vi "K-means Clustering.vi"() -> ()   [LabVIEW 2020]
doc: "The plots display firstly what a K-means algorithm would yield using three clusters. It is then shown what the effect of a bad initialization is on the classification process: By setting n_init to only 1 (default is 10), the amount of times that the algorithm will be run with different centroid seeds is reduced. The next plot displays what using eight clusters would deliver and finally the ground truth."
uses:
  <vilib>/Math Plots/3D Math Plots/3D Scatter/3D Scatter XCtrl/3D Scatter.xctl
  Model/Unsupervised/Cluster/KMeans/KMeans.lvclass
  C:/Users/cipop/TDF Dropbox/2_Technologies de France/1 - Services et Etudes/PLAIY/2 - DEV/PLAIYLAB/code/Model/Model.lvclass
  Model/Unsupervised/Cluster/KMeans/Controls/kmeans_params.ctl
  <vilib>/Math Plots/3D Math Plots/3D Plot/3D Plot Datatype/3D Plot Datatype.lvclass
  PLAIYDISPLAY/Display/_Controls/Style.ctl
  Model/Unsupervised/Cluster/KMeans/KMeans.vi
panel:
  in  "Local":T1
  out "3D Scatter":refnum<class "3D Plot Datatype.lvclass">[](xcontrol)
  out "error out":errorcluster
  in  "error in":errorcluster
  out "3D Scatter 4":refnum<class "3D Plot Datatype.lvclass">[](xcontrol)
  out "3D Scatter 3":refnum<class "3D Plot Datatype.lvclass">[](xcontrol)
  out "3D Scatter 2":refnum<class "3D Plot Datatype.lvclass">[](xcontrol)
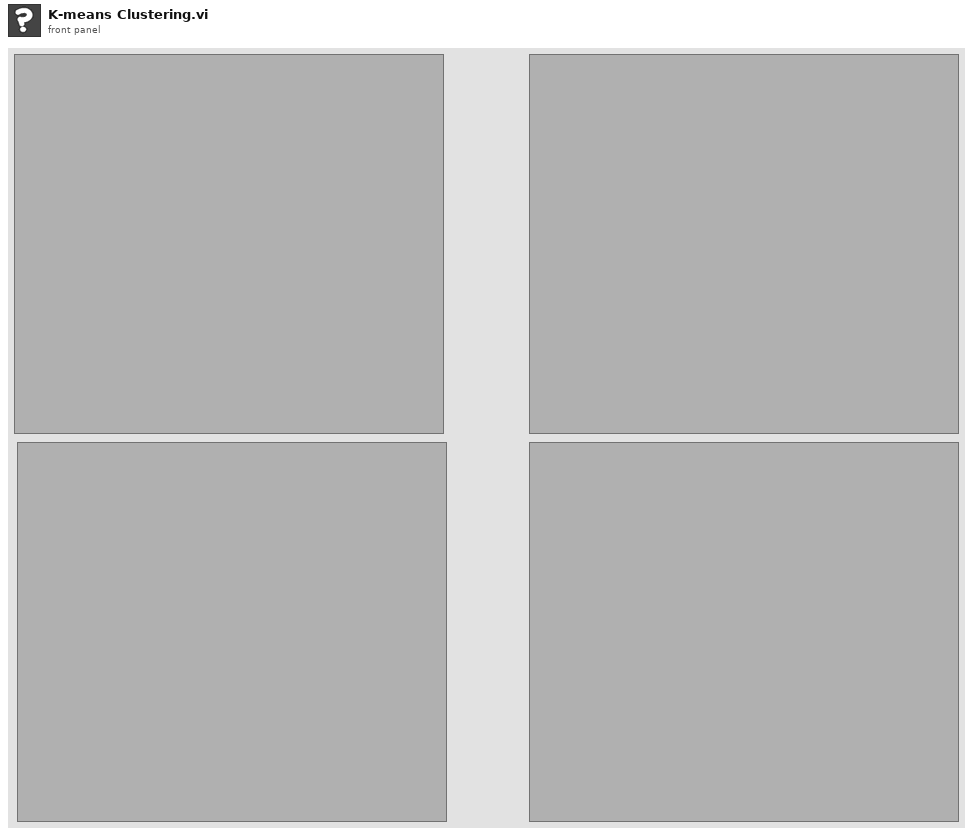
[diagram p1: front panel]
types:
  T1 = cluster{"X":dbl[][], "Y":dbl[], "KMeans":refnum<class "KMeans.lvclass">}
  T2 = typedef "Style.ctl" = enum16{"Empty circle", "Full circle", "Empty square", "Full square", "Cross"}
  T3 = cluster{"Parameter":cluster{"3D Plot":refnum<class "3D Plot Datatype.lvclass">[], "3D Scatter":refnum<vi>, "Data":cluster{"X":dbl[][], "Predict":dbl[][]}, "Display":cluster{"Choice":enum16{"All", "Train", "Test"}, "Indexe":cluster{"X":i32, "Y":i32, "Z":i32}}, "Point Property":cluster{"Style":T2, "Label Color":u32[]}}}
  T4 = typedef "kmeans_params.ctl" = cluster{"n_clusters":dbl, "init":cluster{"init_type":string, "init_list":dbl[][]}, "n_init":dbl, "max_iter":dbl, "tol":dbl, "verbose":dbl, "random_state":dbl, "copy_x":bool, "algorithm":string}
  T5 = typedef "kmeans_attributes.ctl" = cluster{"cluster_centers_":dbl[][], "labels_":dbl[], "inertia_":dbl, "n_iter_":dbl}
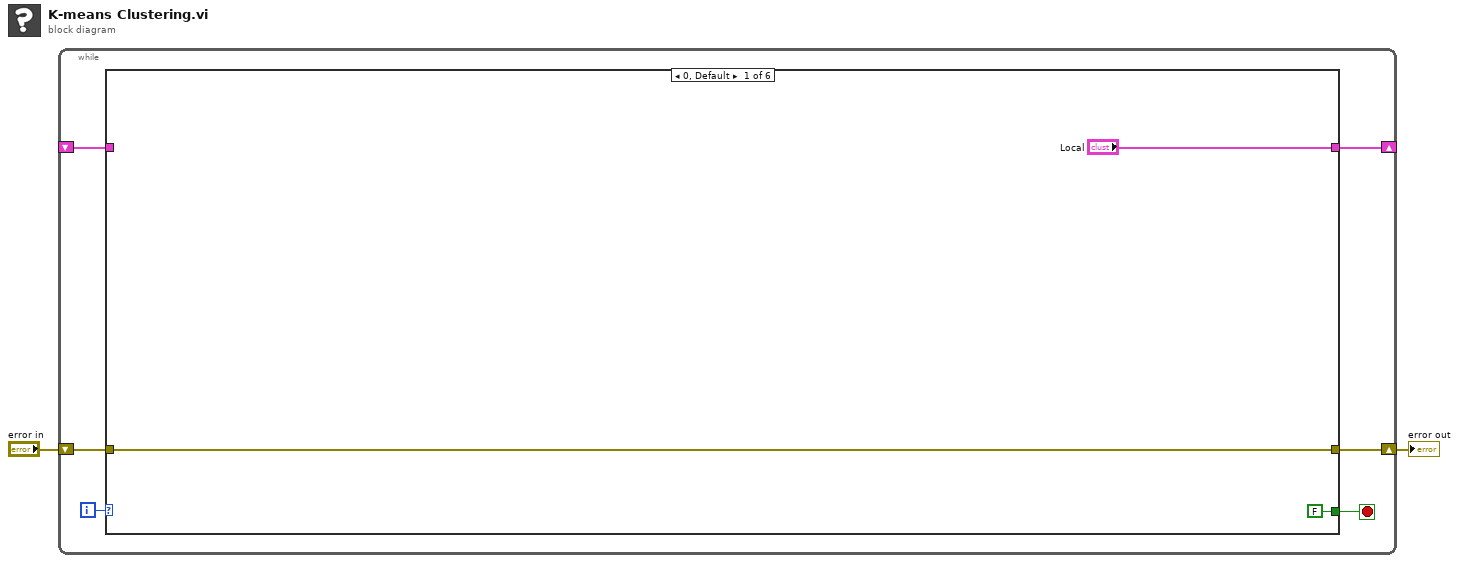
[diagram p0: block diagram]
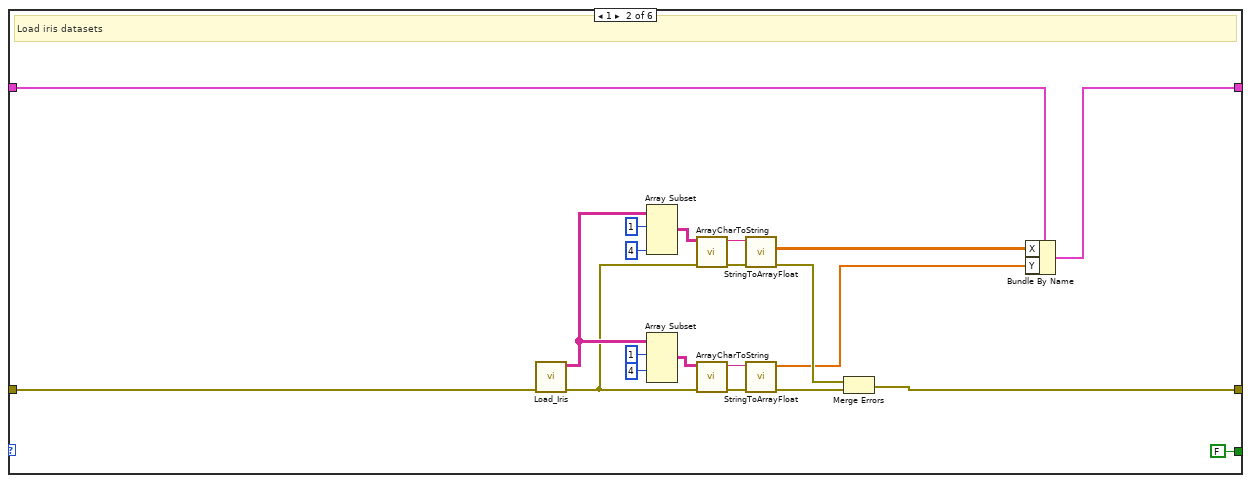
[diagram p2: hidden frame]
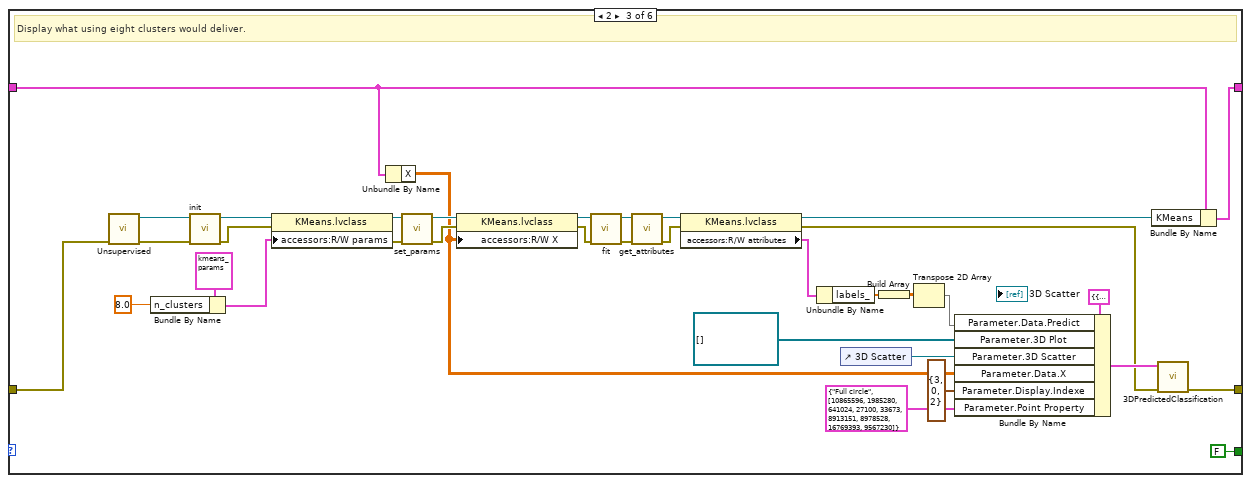
[diagram p3: hidden frame]
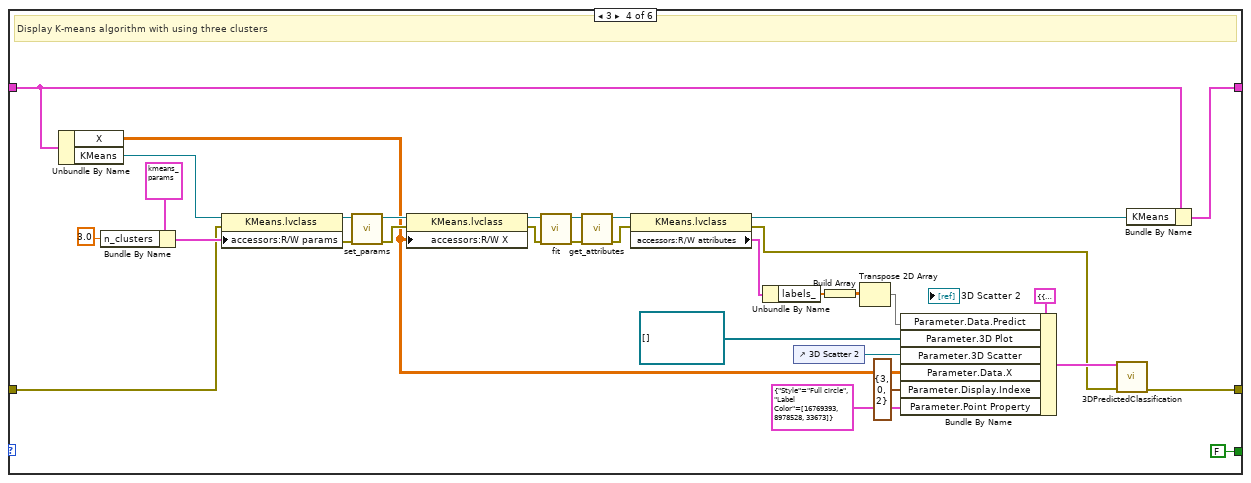
[diagram p4: hidden frame]
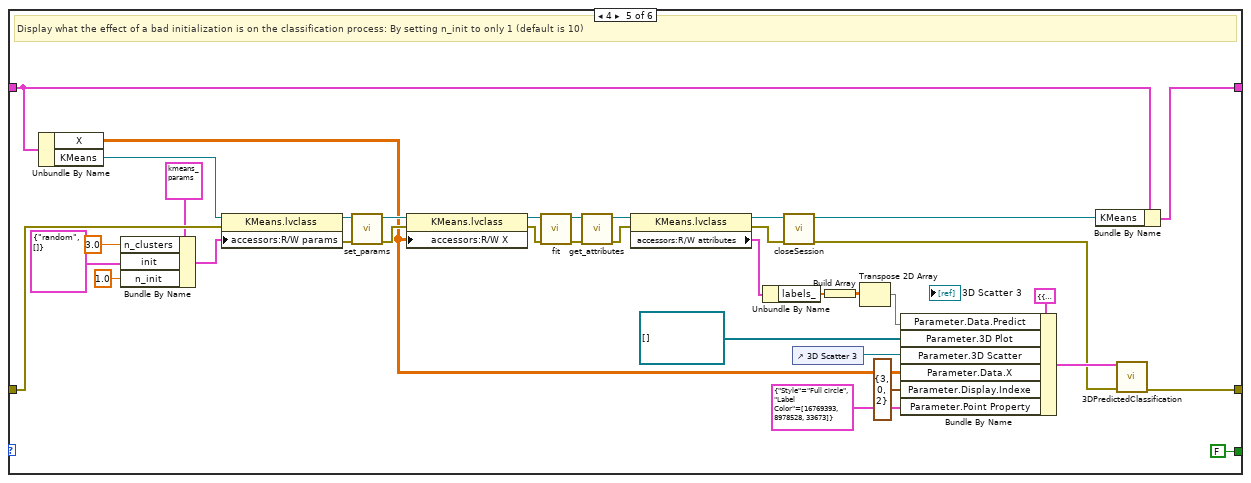
[diagram p5: hidden frame]
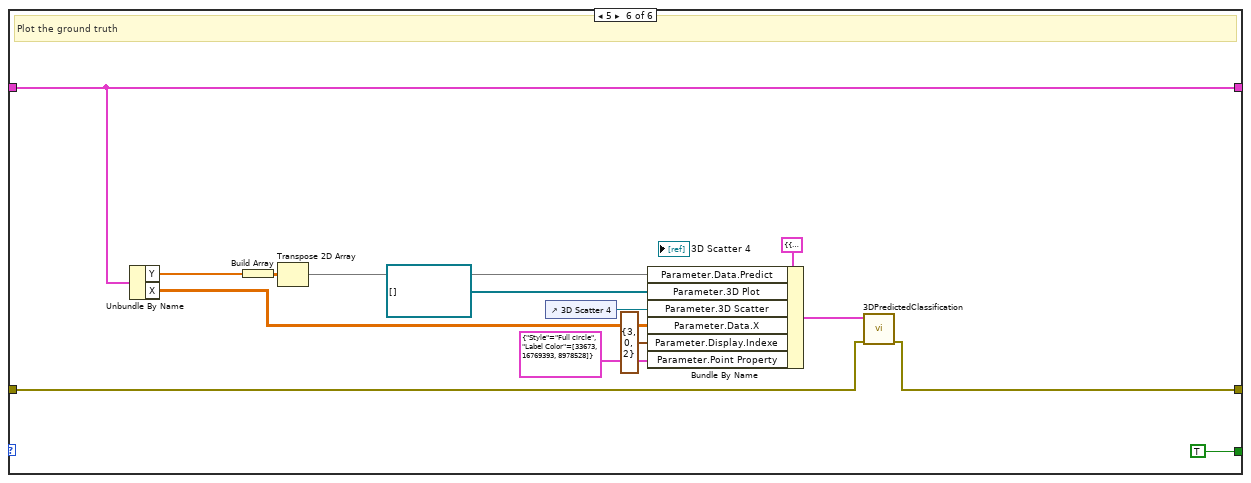
[diagram p6: hidden frame]
diagram:
  n1 = while {
    shift-right: [w6] -> w1
    shift-left: "error in" -> [w7]
    shift-right: [w4] -> _
    shift-left: _ -> [w3]
    i -> [w8]
    stop <- w5 stop-if-true
    n2 = case shown="0, Default" w8 {
      tunnel: w7 -> [w10 w18 w36 w72 w113 w138]
      tunnel: [w10 w17 w37 w75 w114 w139] -> w6
      tunnel: [FALSE FALSE FALSE FALSE FALSE TRUE] -> w5
      tunnel: ["Local" w14 w32 w66 w99 w134] -> w4
      tunnel: w3 -> [_ w15 w33 w68 w100 w134]
      frame 0, Default {
      }
      frame 1 {
        # "Load iris datasets"
        n3 = call "Load_Iris.vi"("error in"=w18) -> ("error out"=w21:errorcluster, "Tableau"=w26:string[][])  [unwired: 9 in]
        n4 = Array Subset(array=w26, index (row)=1 ("index"), length (col)=4 ("length")) -> (w24:string[][])  [unwired: 2 in]
        n5 = Array Subset(array=w26, index (row)=1 ("index"), index (col)=4 ("index")) -> (w22:string[][])  [unwired: 2 in]
        n6 = call "ArrayCharToString.vi"("TAB"=w24) -> ("Instruction"=w25:string)  [unwired: 10 in]
        n7 = call "ArrayCharToString.vi"("TAB"=w22) -> ("Instruction"=w23:string)  [unwired: 10 in]
        n8 = call "StringToArrayFloat.vi"("entrée d'erreur (pas d'erreur)"=w21, "Return value"=w25) -> ("error IO"=w19:errorcluster, "2DArray"=w13:dbl[][])  [unwired: 7 in, 1 out]
        n9 = call "StringToArrayFloat.vi"("entrée d'erreur (pas d'erreur)"=w21, "Return value"=w23) -> ("error IO"=w20:errorcluster, "1DArray"=w12:dbl[])  [unwired: 7 in, 1 out]
        n10 = Merge Errors(w19, w20) -> (w17:errorcluster)
        n11 = Bundle By Name(cluster=w15, "X"=w13, "Y"=w12) -> (w14:T1)
      }
      frame 2 {
        # "Display what using eight clusters would deliver."
        n12 = call-poly "Unsupervised.vi"("error in"=w36) -> ("error out"=w57:errorcluster, "out"=w58:refnum<class "KMeans.lvclass">)  [unwired: 9 in]
        n13 = Bundle By Name(cluster=T4 {"n_clusters"=8.0, "init"={"init_type"="k-means++", "init_list"=[]}, "n_init"=10.0, "max_iter"=300.0, "tol"=0.0001, "verbose"=0.0, "random_state"=0.0, "copy_x"=TRUE, "algorithm"="auto"} ("R/W params"), "n_clusters"=8.0) -> (w59:T4)
        n14 = call-dynamic "init.vi"("error in (no error)"=w57, "Model en entrée"=w58) -> ("error out"=w60:errorcluster, "Model en sortie"=w64:refnum<class "KMeans.lvclass">)  [unwired: 8 in]
        n15 = property class="KMeans.lvclass"(reference=w64, error in=w60, "accessors:R/W params"=w59) -> (reference out=w63:refnum<class "KMeans.lvclass">, error out=w65:errorcluster)
        n16 = Unbundle By Name(w33) -> ("X"=w34:dbl[][])
        n17 = call-dynamic "set_params.vi"("error in (no error)"=w65, "KMeans.lvclass 2"=w63) -> ("error out"=w61:errorcluster, "KMeans.lvclass"=w62:refnum<class "KMeans.lvclass">)  [unwired: 8 in]
        n18 = property class="KMeans.lvclass"(reference=w62, error in=w61, "accessors:R/W X"=w34) -> (reference out=w55:refnum<class "KMeans.lvclass">, error out=w54:errorcluster)
        n19 = call-dynamic "fit.vi"("error in (no error)"=w54, "KMeans.lvclass 2"=w55) -> ("error out"=w50:errorcluster, "KMeans.lvclass"=w51:refnum<class "KMeans.lvclass">)  [unwired: 8 in]
        n20 = call-dynamic "get_attributes.vi"("error in (no error)"=w50, "KMeans.lvclass 2"=w51) -> ("error out"=w52:errorcluster, "KMeans.lvclass"=w53:refnum<class "KMeans.lvclass">)  [unwired: 8 in]
        n21 = property class="KMeans.lvclass"(reference=w53, error in=w52) -> (reference out=w31:refnum<class "KMeans.lvclass">, error out=w39:errorcluster, "accessors:R/W attributes"=w47:T5)
        n22 = Unbundle By Name(w47) -> ("labels_"=w46:dbl[])
        n23 = control-ref of="3D Scatter"() -> (w40:refnum<vi>)
        n24 = Build Array(w46) -> (w42:dbl[][])
        n25 = Transpose 2D Array(2D array=w42) -> (transposed array=w41:dbl[][])
        n26 = Bundle By Name(cluster=T3 {"Parameter"={"3D Plot"=[], "3D Scatter"=refnum, "Data"={"X"=[], "Predict"=[]}, "Display"={"Choice"=enum."All", "Indexe"={"X"=0, "Y"=1, "Z"=2}}, "Point Property"={"Style"=enum."Full circle", "Label Color"=[8978528, 4367871, 1985280]}}} ("Parameters"), "Parameter.Data.Predict"=w41, "Parameter.3D Plot"=refnum<class "3D Plot Datatype.lvclass">[] [] ("3D Scatter"), "Parameter.3D Scatter"=w40, "Parameter.Data.X"=w34, "Parameter.Display.Indexe"=cluster{"X":i32, "Y":i32, "Z":i32} {"X"=3, "Y"=0, "Z"=2}, "Parameter.Point Property"=cluster{"Style":T2, "Label Color":u32[]} {"Style"=enum."Full circle", "Label Color"=[10865596, 1985280, 641024, 27100, 33673, 8913151, 8978528, 16769393, 9567230]} ("Point Property")) -> (w43:T3)
        n27 = Bundle By Name(cluster=w33, "KMeans"=w31) -> (w32:T1)
        n28 = call "3DPredictedClassification.vi"("error in"=w39, "Parameters"=w43) -> ("error out"=w37:errorcluster)  [unwired: 8 in, 1 out]
      }
      frame 3 {
        # "Display K-means algorithm with using three clusters"
        n29 = Unbundle By Name(w68) -> ("X"=w70:dbl[][], "KMeans"=w69:refnum<class "KMeans.lvclass">)
        n30 = Bundle By Name(cluster=T4 {"n_clusters"=8.0, "init"={"init_type"="k-means++", "init_list"=[]}, "n_init"=10.0, "max_iter"=300.0, "tol"=0.0001, "verbose"=0.0, "random_state"=0.0, "copy_x"=TRUE, "algorithm"="auto"} ("R/W params"), "n_clusters"=3.0) -> (w73:T4)
        n31 = property class="KMeans.lvclass"(reference=w69, error in=w72, "accessors:R/W params"=w73) -> (reference out=w89:refnum<class "KMeans.lvclass">, error out=w88:errorcluster)
        n32 = call-dynamic "set_params.vi"("error in (no error)"=w88, "KMeans.lvclass 2"=w89) -> ("error out"=w91:errorcluster, "KMeans.lvclass"=w90:refnum<class "KMeans.lvclass">)  [unwired: 8 in]
        n33 = property class="KMeans.lvclass"(reference=w90, error in=w91, "accessors:R/W X"=w70) -> (reference out=w92:refnum<class "KMeans.lvclass">, error out=w93:errorcluster)
        n34 = call-dynamic "fit.vi"("error in (no error)"=w93, "KMeans.lvclass 2"=w92) -> ("error out"=w97:errorcluster, "KMeans.lvclass"=w96:refnum<class "KMeans.lvclass">)  [unwired: 8 in]
        n35 = call-dynamic "get_attributes.vi"("error in (no error)"=w97, "KMeans.lvclass 2"=w96) -> ("error out"=w95:errorcluster, "KMeans.lvclass"=w94:refnum<class "KMeans.lvclass">)  [unwired: 8 in]
        n36 = property class="KMeans.lvclass"(reference=w94, error in=w95) -> (reference out=w67:refnum<class "KMeans.lvclass">, error out=w77:errorcluster, "accessors:R/W attributes"=w79:T5)
        n37 = Unbundle By Name(w79) -> ("labels_"=w82:dbl[])
        n38 = control-ref of="3D Scatter 2"() -> (w76:refnum<vi>)
        n39 = Build Array(w82) -> (w85:dbl[][])
        n40 = Transpose 2D Array(2D array=w85) -> (transposed array=w86:dbl[][])
        n41 = Bundle By Name(cluster=T3 {"Parameter"={"3D Plot"=[], "3D Scatter"=refnum, "Data"={"X"=[], "Predict"=[]}, "Display"={"Choice"=enum."All", "Indexe"={"X"=0, "Y"=1, "Z"=2}}, "Point Property"={"Style"=enum."Full circle", "Label Color"=[8978528, 4367871, 1985280]}}} ("Parameters"), "Parameter.Data.Predict"=w86, "Parameter.3D Plot"=refnum<class "3D Plot Datatype.lvclass">[] [] ("3D Scatter"), "Parameter.3D Scatter"=w76, "Parameter.Data.X"=w70, "Parameter.Display.Indexe"=cluster{"X":i32, "Y":i32, "Z":i32} {"X"=3, "Y"=0, "Z"=2}, "Parameter.Point Property"=cluster{"Style":T2, "Label Color":u32[]} {"Style"=enum."Full circle", "Label Color"=[16769393, 8978528, 33673]} ("Point Property")) -> (w78:T3)
        n42 = call "3DPredictedClassification.vi"("error in"=w77, "Parameters"=w78) -> ("error out"=w75:errorcluster)  [unwired: 8 in, 1 out]
        n43 = Bundle By Name(cluster=w68, "KMeans"=w67) -> (w66:T1)
      }
      frame 4 {
        # "Display what the effect of a bad initialization is on the classification process: By setting n_init to only 1 (default is 10)"
        n44 = Unbundle By Name(w100) -> ("X"=w102:dbl[][], "KMeans"=w101:refnum<class "KMeans.lvclass">)
        n45 = Bundle By Name(cluster=T4 {"n_clusters"=8.0, "init"={"init_type"="k-means++", "init_list"=[]}, "n_init"=10.0, "max_iter"=300.0, "tol"=0.0001, "verbose"=0.0, "random_state"=0.0, "copy_x"=TRUE, "algorithm"="auto"} ("R/W params"), "n_clusters"=3.0, "init"=cluster{"init_type":string, "init_list":dbl[][]} {"init_type"="random", "init_list"=[]}, "n_init"=1.0) -> (w108:T4)
        n46 = property class="KMeans.lvclass"(reference=w101, error in=w113, "accessors:R/W params"=w108) -> (reference out=w125:refnum<class "KMeans.lvclass">, error out=w124:errorcluster)
        n47 = call-dynamic "set_params.vi"("error in (no error)"=w124, "KMeans.lvclass 2"=w125) -> ("error out"=w127:errorcluster, "KMeans.lvclass"=w126:refnum<class "KMeans.lvclass">)  [unwired: 8 in]
        n48 = property class="KMeans.lvclass"(reference=w126, error in=w127, "accessors:R/W X"=w102) -> (reference out=w128:refnum<class "KMeans.lvclass">, error out=w129:errorcluster)
        n49 = call-dynamic "fit.vi"("error in (no error)"=w129, "KMeans.lvclass 2"=w128) -> ("error out"=w133:errorcluster, "KMeans.lvclass"=w132:refnum<class "KMeans.lvclass">)  [unwired: 8 in]
        n50 = call-dynamic "get_attributes.vi"("error in (no error)"=w133, "KMeans.lvclass 2"=w132) -> ("error out"=w131:errorcluster, "KMeans.lvclass"=w130:refnum<class "KMeans.lvclass">)  [unwired: 8 in]
        n51 = property class="KMeans.lvclass"(reference=w130, error in=w131) -> (reference out=w106:refnum<class "KMeans.lvclass">, error out=w105:errorcluster, "accessors:R/W attributes"=w116:T5)
        n52 = Unbundle By Name(w116) -> ("labels_"=w119:dbl[])
        n53 = call-dynamic "closeSession.vi"("error in"=w105, "Python en entrée"=w106) -> ("error out"=w104:errorcluster, "Python en sortie"=w98:refnum<class "KMeans.lvclass">)  [unwired: 8 in]
        n54 = control-ref of="3D Scatter 3"() -> (w107:refnum<vi>)
        n55 = Build Array(w119) -> (w122:dbl[][])
        n56 = Transpose 2D Array(2D array=w122) -> (transposed array=w123:dbl[][])
        n57 = Bundle By Name(cluster=T3 {"Parameter"={"3D Plot"=[], "3D Scatter"=refnum, "Data"={"X"=[], "Predict"=[]}, "Display"={"Choice"=enum."All", "Indexe"={"X"=0, "Y"=1, "Z"=2}}, "Point Property"={"Style"=enum."Full circle", "Label Color"=[8978528, 4367871, 1985280]}}} ("Parameters"), "Parameter.Data.Predict"=w123, "Parameter.3D Plot"=refnum<class "3D Plot Datatype.lvclass">[] [] ("3D Scatter"), "Parameter.3D Scatter"=w107, "Parameter.Data.X"=w102, "Parameter.Display.Indexe"=cluster{"X":i32, "Y":i32, "Z":i32} {"X"=3, "Y"=0, "Z"=2}, "Parameter.Point Property"=cluster{"Style":T2, "Label Color":u32[]} {"Style"=enum."Full circle", "Label Color"=[16769393, 8978528, 33673]} ("Point Property")) -> (w115:T3)
        n58 = Bundle By Name(cluster=w100, "KMeans"=w98) -> (w99:T1)
        n59 = call "3DPredictedClassification.vi"("error in"=w104, "Parameters"=w115) -> ("error out"=w114:errorcluster)  [unwired: 8 in, 1 out]
      }
      frame 5 {
        # "Plot the ground truth"
        n60 = Unbundle By Name(w134) -> ("Y"=w136:dbl[], "X"=w135:dbl[][])
        n61 = Build Array(w136) -> (w142:dbl[][])
        n62 = Transpose 2D Array(2D array=w142) -> (transposed array=w140:dbl[][])
        n63 = control-ref of="3D Scatter 4"() -> (w141:refnum<vi>)
        n64 = Bundle By Name(cluster=T3 {"Parameter"={"3D Plot"=[], "3D Scatter"=refnum, "Data"={"X"=[], "Predict"=[]}, "Display"={"Choice"=enum."All", "Indexe"={"X"=0, "Y"=1, "Z"=2}}, "Point Property"={"Style"=enum."Full circle", "Label Color"=[8978528, 4367871, 1985280]}}} ("Parameters"), "Parameter.Data.Predict"=w140, "Parameter.3D Plot"=refnum<class "3D Plot Datatype.lvclass">[] [] ("3D Scatter"), "Parameter.3D Scatter"=w141, "Parameter.Data.X"=w135, "Parameter.Display.Indexe"=cluster{"X":i32, "Y":i32, "Z":i32} {"X"=3, "Y"=0, "Z"=2}, "Parameter.Point Property"=cluster{"Style":T2, "Label Color":u32[]} {"Style"=enum."Full circle", "Label Color"=[33673, 16769393, 8978528]} ("Point Property")) -> (w144:T3)
        n65 = call "3DPredictedClassification.vi"("error in"=w138, "Parameters"=w144) -> ("error out"=w139:errorcluster)  [unwired: 8 in, 1 out]
      }
    }
  }
  "error out" <- w1
